vi "Graph Child.vi"() -> ()   [LabVIEW 2014]
panel:
  in  "Events Registered":T1
  in  "error in (no error)":errorcluster
  in  "User Events VR":variant
  out "Waveform Chart":dbl(graph)
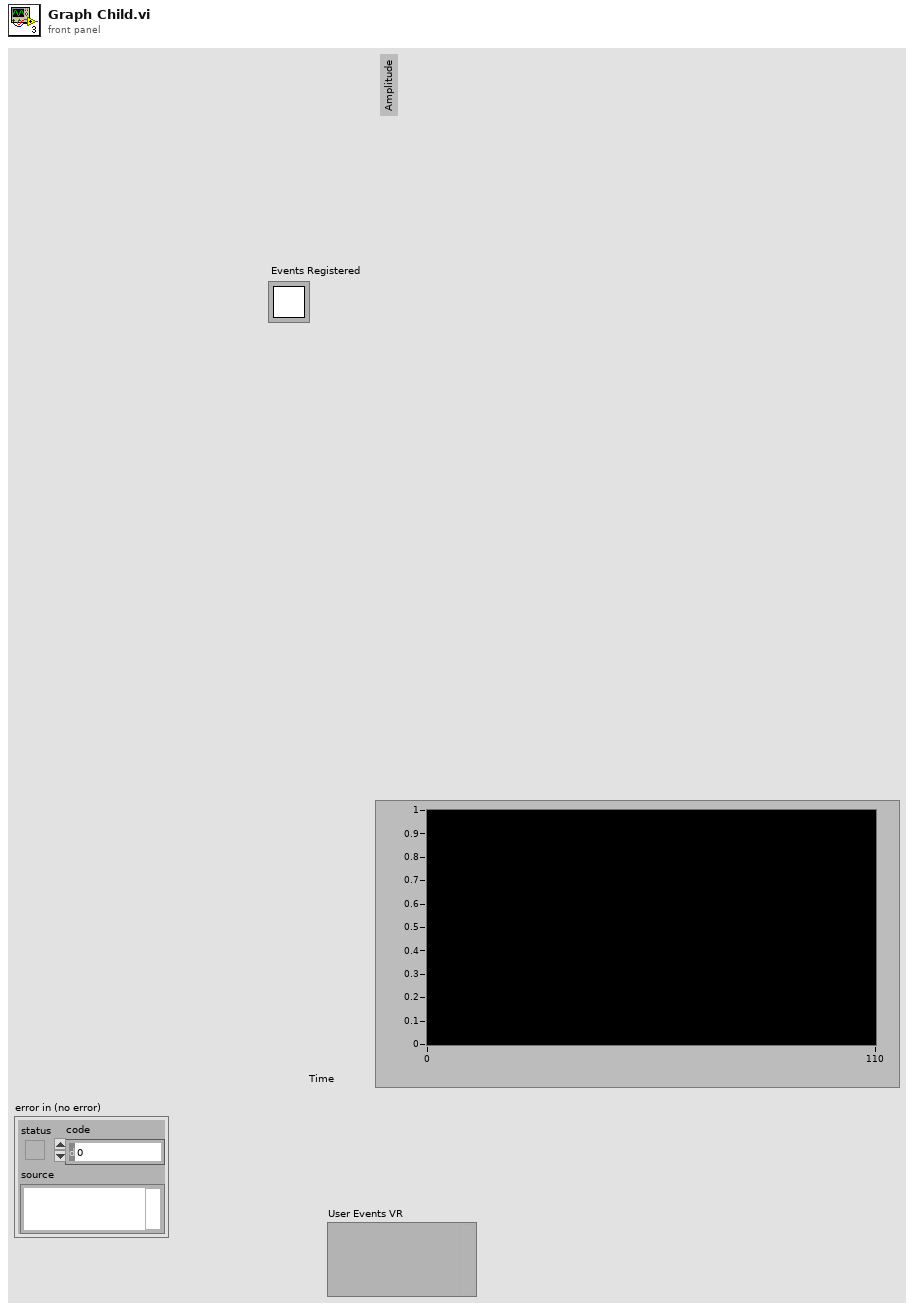
[diagram p1: front panel]
types:
  T1 = typedef "Semaphore RefNum" = refnum<k1>
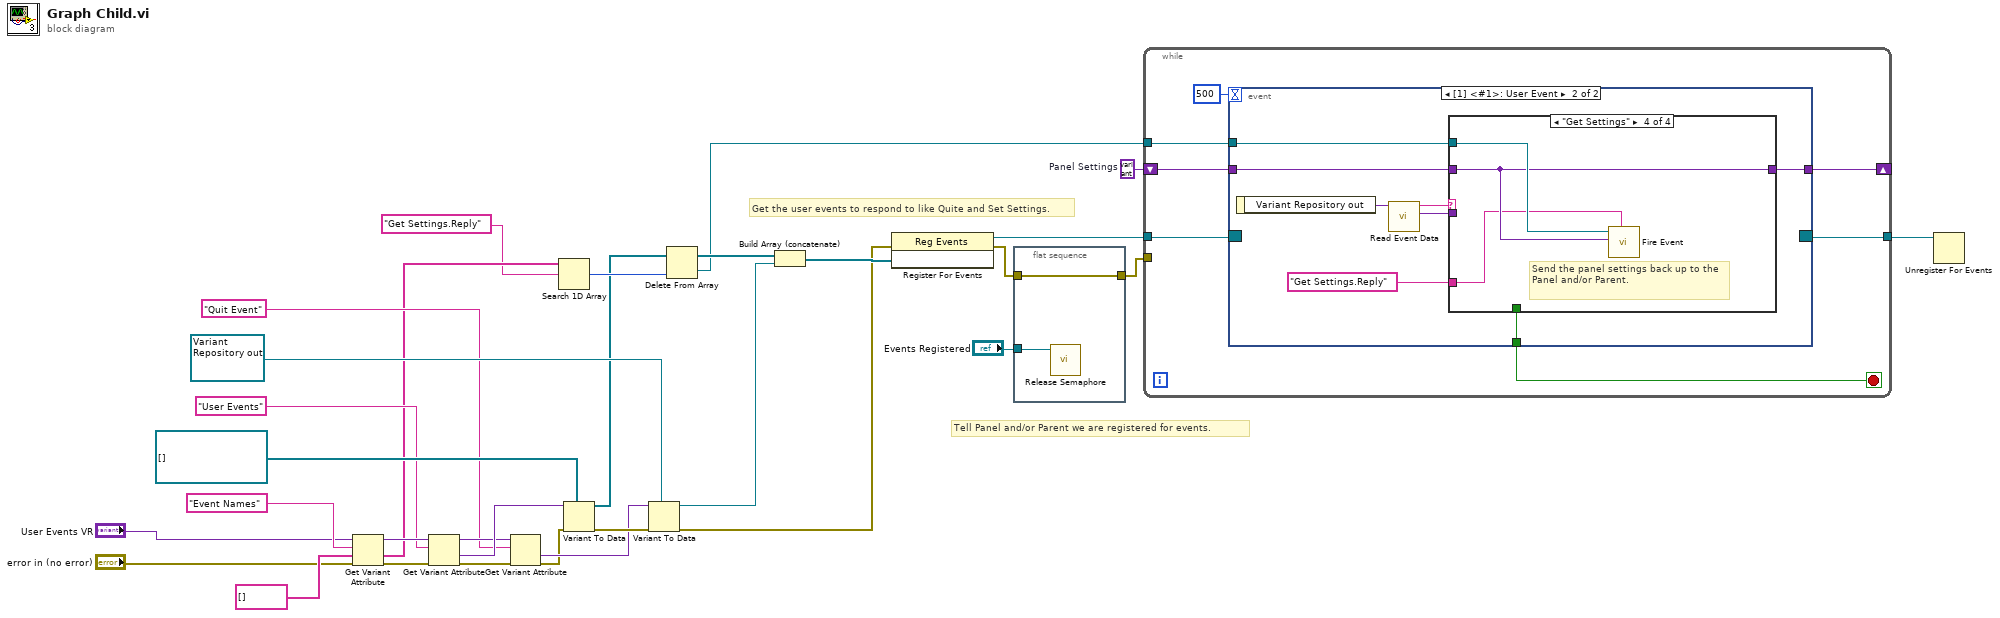
[diagram p0: block diagram]
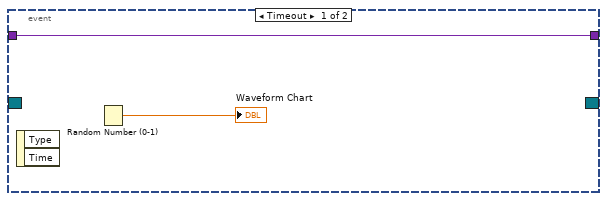
[diagram p2: hidden frame]
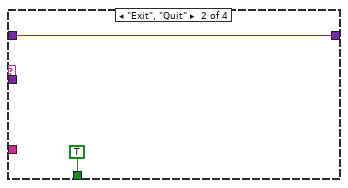
[diagram p4: hidden frame]
diagram:
  w27 = variant  # Panel Settings
  # "Get the user events to respond to like Quite and Set Settings."
  # "Tell Panel and/or Parent we are registered for events."
  n1 = Get Variant Attribute(Variant="User Events VR", name="Event Names" ("Tag"), default value (empty Variant)=string[] [], error in="error in (no error)") -> (duplicate Variant=w16:variant, value=w5:string[], error out=w15:errorcluster)  [unwired: 1 out]
  n2 = Get Variant Attribute(Variant=w16, name="User Events" ("Tag"), error in=w15) -> (duplicate Variant=w12:variant, value=w13:variant, error out=w11:errorcluster)  [unwired: 1 in, 1 out]
  n3 = Get Variant Attribute(Variant=w12, name="Quit Event" ("Tag"), error in=w11) -> (value=w9:variant, error out=w8:errorcluster)  [unwired: 1 in, 2 out]
  n4 = Search 1D Array(1D array=w5, element="Get Settings.Reply") -> (index of element=w26:i32)  [unwired: 1 in]
  n5 = Variant To Data(error in=w8, type=refnum<user-event>[] [] ("All User Events"), Variant=w13) -> (data=w4:refnum<user-event>[], error out=w19:errorcluster)
  n6 = Variant To Data(error in=w19, type=refnum<user-event> refnum ("Quit Event"), Variant=w9) -> (data=w3:refnum<user-event>, error out=w2:errorcluster)
  n7 = Delete From Array(array=w4, index=w26) -> (deleted portion=w23:refnum<user-event>, array with subset deleted=w25:refnum<user-event>[])  [unwired: 1 in]
  n8 = Build Array (concatenate)(w25, w3) -> (w24:refnum<user-event>[])
  n9 = register-events(error in=w2, w24) -> (reference out=w31:refnum<event-registration>, error out=w29:errorcluster)  [unwired: 1 in]
  n10 = flat-sequence {
    tunnel: w29 -> [w33]
    tunnel: [w33] -> w28
    tunnel: "Events Registered" -> [w32]
    frame #0 {
      n11 = call <vilib>:"Release Semaphore.vi"("semaphore"=w32) -> ()  [unwired: 5 in, 2 out]
    }
  }
  n12 = while {
    tunnel: w31 -> [w39]
    tunnel: [w37] -> w30
    tunnel: w28 -> [_]
    shift-right: [w36] -> _
    shift-left: w27 -> [w35]
    tunnel: w23 -> [w34]
    stop <- w38 stop-if-true
    n13 = event shown="[1] <#1>: User Event" {
      selector: w39 -> [_ _]
      dyn-events: [_ _] -> w37
      timeout: 500 -> [_ _]
      tunnel: [_ w48] -> w38
      tunnel: [w41 w46] -> w36
      tunnel: w35 -> [w41 w45]
      tunnel: w34 -> [_ w44]
      event Timeout {
        n14 = event-data() -> ()  [unwired: 1 in, 2 out]
        n15 = Random Number (0-1)() -> (number: 0 to 1=→"Waveform Chart":dbl)
      }
      event User Event {
        n16 = event-data() -> ("Variant Repository out"=w50:variant)  [unwired: 1 in]
        n17 = call "Read Event Data.vi"("Variant Data"=w50) -> ("Event Data"=w47:variant, "Event Name"=w49:string)  [unwired: 8 in, 1 out]
        n18 = case shown="\"Get Settings\"" w49 {
          tunnel: [_ TRUE _ _] -> w48
          tunnel: w47 -> [_ _ w54 _]
          tunnel: [w51 w52 w54 w56] -> w46
          tunnel: w45 -> [w51 w52 _ w56]
          tunnel: w44 -> [_ _ _ w57]
          tunnel: "Get Settings.Reply" ("element") -> [_ _ _ w55]
          frame Default {
          }
          frame "Exit", "Quit" {
          }
          frame "Set Settings" {
            # "Take the settings and apply them, here we can have a set of steps to perform like clearing the graph, and registering for data to display."
          }
          frame "Get Settings" {
            # "Send the panel settings back up to the Panel and/or Parent."
            n19 = call "Fire Event.vi"("Event Name"=w55, "Event Data"=w56, "User Event In"=w57) -> ()  [unwired: 7 in, 2 out]
          }
        }
      }
    }
  }
  n20 = Unregister For Events(event registration refnum=w30) -> ()  [unwired: 1 in, 1 out]
